vi "Renishaw-XL80_SetFastAveraging.vi"(8 "error in (no error)":errorcluster, 11 "Renishaw-XL80 in":refnum<class "Renishaw-XL80.lvclass">) -> (0 "error out":errorcluster, 3 "Renishaw-XL80 out":refnum<class "Renishaw-XL80.lvclass">)   [LabVIEW 2024, in "Renishaw-XL80.lvclass"]
doc: "This method will set short-term averaging of the ML10 reading on.\n\nDefinition\nHRESULTSetSlowAveraging();\nParameters\nNone\n\nComments\nThis method will return with an HRESULT of E_FAIL if the client has not previously connected to a DX10 by calling Connect. The method will also return E_FAIL if the DX10 is not responding or the ML10 is not responding. Otherwise the method will return an HRESULT of S_OK.\n\nShort term (fast) averaging enables a \"box car\" averaging algorithm inside the ML10 with a response time of approximately 1/4sec.\n\nNote that short term averaging is on when the ML10 status has ML10_AVERAGING_ON set and ML10_LONG_TERM_AVERAGING_ON not set.\n\nNote that averaging has no effect on synchronous TPin triggered readings."
uses:
  Renishaw-XL80.lvclass
  Renishaw-XL80.lvclass/Renishaw-XL80.ctl
  D:/A.C.M/Example CSharp_64/bin/Debug/Interop.DX10SDKADAPTORLib.dll
  Example CSharp_64/bin/Debug/Interop.DX10SDKADAPTORLib.dll
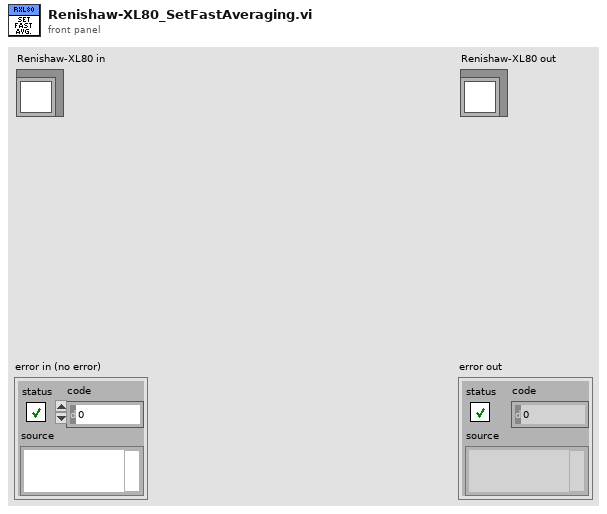
[diagram p1: front panel]
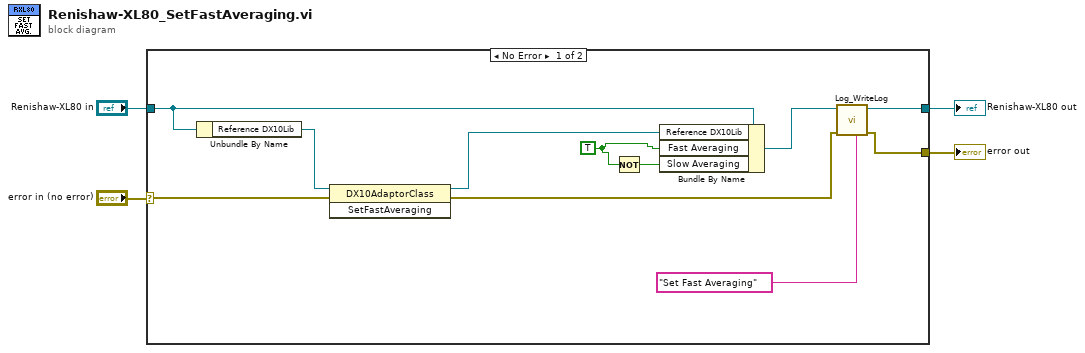
[diagram p0: block diagram]
diagram:
  n1 = case shown="No Error" "error in (no error)" {
    selector: "error in (no error)" -> [w14 w17]
    tunnel: [w10 w17] -> w3
    tunnel: [w12 w16] -> w1
    tunnel: "Renishaw-XL80 in" -> [w13 w16]
    frame No Error {
      w5 = TRUE ("Fast Averaging")
      n2 = Unbundle By Name(w13) -> ("Reference DX10Lib"=w15:refnum<k24>)
      n3 = invoke class="DX10AdaptorClass" method="SetFastAveraging"(reference=w15, error in=w14) -> (reference out=w9:refnum<k24>, error out=w8:errorcluster)  [unwired: 1 in, 1 out]
      n4 = Not(x=w5) -> (.not. x?=w6:bool)
      n5 = Bundle By Name(cluster=w13, "Reference DX10Lib"=w9, "Fast Averaging"=w5, "Slow Averaging"=w6) -> (w11:refnum<class "Renishaw-XL80.lvclass">)
      n6 = call-dynamic "Log_WriteLog.vi"("Additional text"="Set Fast Averaging", "error in (no error)"=w8, "Log in"=w11) -> ("error out"=w10:errorcluster, "Log out"=w12:refnum<class "Renishaw-XL80.lvclass">)  [unwired: 7 in]
    }
    frame Error {
    }
  }
  "error out" <- w3
  "Renishaw-XL80 out" <- w1
